vi "Disconnect.vi"(8 "error in (no error)":errorcluster, 11 "reference in":refnum<class "NS slave.lvclass">) -> (0 "error out":errorcluster, 3 "reference out":refnum<class "NS slave.lvclass">)   [LabVIEW 2019, in "CommandResponse communication.lvlib" / "NS slave.lvclass"]
doc: "Close all network streams to slave"
uses:
  NS slave.lvclass
  C:/Barkhausen mmWave radar/Development/LV/Barkhausen mmWave hardware control/Host/Intertarget communication/CR slave_class/CR slave.lvclass
  ITC command.ctl
  ITC response.ctl
  CommandResponse communication.lvlib
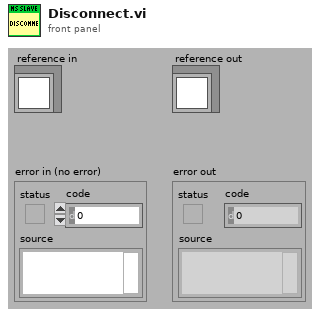
[diagram p1: front panel]
types:
  T1 = typedef "CommandResponse communication.lvlib/NS slave.lvclass/ObjectAttributesRef.ctl" = refnum<data-value>
  T2 = typedef "CommandResponse communication.lvlib/NS slave.lvclass/ObjectAttributes.ctl" = cluster{"connected":bool, "stop":bool, "ID":string, "command rd":refnum<k21>, "response wr":refnum<k21>, "data wr":refnum<k21>}
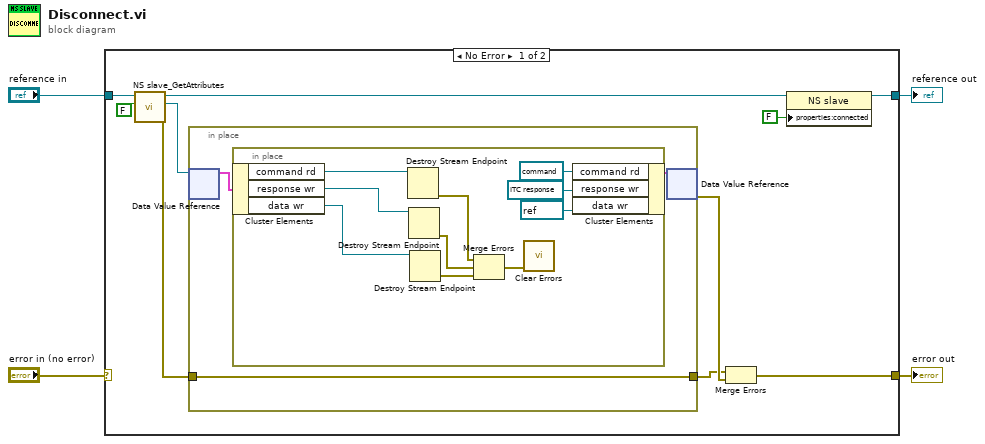
[diagram p0: block diagram]
diagram:
  n1 = case shown="No Error" "error in (no error)" {
    selector: "error in (no error)" -> [_ w29]
    tunnel: [w14 w29] -> w3
    tunnel: [w6 w28] -> w1
    tunnel: "reference in" -> [w11 w28]
    frame No Error {
      n2 = call "NS slave_GetAttributes.vi"("return data? (T)"=FALSE, "reference in"=w11) -> ("error out"=w9:errorcluster, "attributes ref"=w7:T1, "reference out"=w8:refnum<class "NS slave.lvclass">)  [unwired: 6 in, 1 out]
      n3 = in-place {
        in-place-border: w9 -> [w15]
        in-place-border: [w15] -> w12
        n4 = in-place-dvr #1(w7) -> (w16:T2)  [unwired: 1 out]
        n5 = in-place {
          n6 = in-place-cluster #2(w16) -> ("command rd"=w27:refnum<k21>, "response wr"=w26:refnum<k21>, "data wr"=w25:refnum<k21>)
          n7 = Destroy Stream Endpoint(11:w27) -> (0:w23:errorcluster)  [unwired: 1 in]
          n8 = Destroy Stream Endpoint(11:w26) -> (0:w22:errorcluster)  [unwired: 1 in]
          n9 = Destroy Stream Endpoint(11:w25) -> (0:w24:errorcluster)  [unwired: 1 in]
          n10 = Merge Errors(w23, w22, w24) -> (w21:errorcluster)
          n11 = call <vilib>:"Clear Errors.vi"("error in (no error)"=w21) -> ()  [unwired: 5 in, 2 out]
          n12 = in-place-cluster #2("command rd"=refnum<k21> refnum, "response wr"=refnum<k21> refnum, "data wr"=refnum<k21> refnum) -> (w17:T2)
        }
        n13 = in-place-dvr #1(w17) -> (w13:errorcluster)  [unwired: 1 out]
      }
      n14 = Merge Errors(w12, w13) -> (w14:errorcluster)
      n15 = property class="NS slave"(reference=w8, "properties:connected"=FALSE ("connected")) -> (reference out=w6:refnum<class "NS slave.lvclass">)  [unwired: 1 in, 1 out]
    }
    frame Error {
    }
  }
  "error out" <- w3
  "reference out" <- w1
